vi "Config Retrigger.vi"(0 "VISA Resource Name":refnum<visa-resource-name>, 5 "Standard (0: IS-95A)":T1(ring), 7 "State (T: ON)":bool=TRUE, 11 "error in (no error)":errorcluster {"code" format="%.0x"}) -> (4 "VISA Resource Name Out":refnum<visa-resource-name>, 15 "error out":errorcluster {"code" format="%.0x"})   [LabVIEW 2012, in "Agilent ESG Series.lvlib"]
doc: "This VI enables or disables the ARB retriggering mode; the retrigger mode controls how the retriggering function performs while a waveform is playing."
uses:
  <instrlib>/Agilent ESG Series/Agilent ESG Series.lvlib
panel:
  # "ON"
  # "OFF"
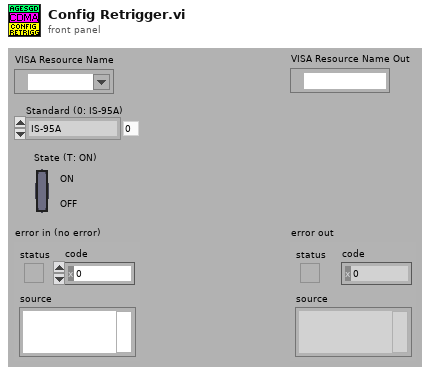
[diagram p1: front panel]
types:
  T1 = enum16{"IS-95A", "CDMA2000", "WCDMA", "Dual Arbitrary"}
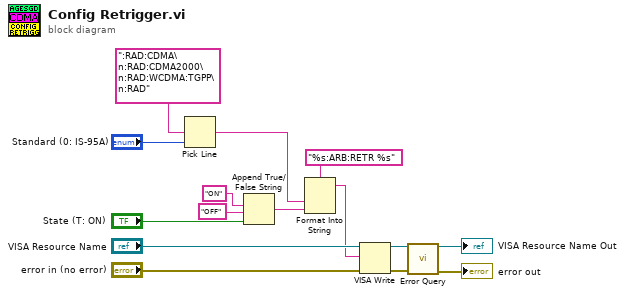
[diagram p0: block diagram]
diagram:
  n1 = Pick Line(multi-line string=":RAD:CDMA\n:RAD:CDMA2000\n:RAD:WCDMA:TGPP\n:RAD", line index="Standard (0: IS-95A)") -> (output string=w8:string)  [unwired: 1 in]
  n2 = Append True/False String(1:"State (T: ON)", 2:"OFF" ("false string"), 3:"ON" ("multi-line string")) -> (0:w2:string)  [unwired: 1 in]
  n3 = Format Into String(format string="%s:ARB:RETR %s", w8, w2) -> (resulting string=w1:string)  [unwired: 2 in, 1 out]
  n4 = VISA Write(VISA resource name="VISA Resource Name", write buffer=w1, error in (no error)="error in (no error)") -> (VISA resource name out=w11:refnum<visa-resource-name>, error out=w10:errorcluster)  [unwired: 1 out]
  n5 = call <instrlib>:"Error Query.vi"("VISA Resource Name"=w11, "error in (no error)"=w10) -> ("VISA Resource Name Out"=→"VISA Resource Name Out":refnum<visa-resource-name>, "error out"=→"error out":errorcluster)  [unwired: 10 in, 2 out]
